vi "DestroyAllSessions.vi"(7 "DLL path":path, 8 "error in (no error)":errorcluster) -> (0 "error out":errorcluster)   [LabVIEW 2017, in "ONNX Class Library.lvlib"]
doc: "/**\n * @brief Уничтожить ВСЕ активные сессии (полная очистка памяти)\n * \n * Эта функция находит все созданные сессии в хранилище, освобождает их память,\n * удаляет метаданные и очищает список сессий. Полезно вызывать при завершении\n * работы приложения для гарантированного освобождения ресурсов.\n * \n * @return void\n * \n * @note После вызова все ранее полученные SessionID становятся невалидными\n * @note Не нужно вызывать DestroySession для каждой сессии отдельно\n * @note Безопасно вызывать, даже если сессий не было создано (ничего не сделает)\n */\nvoid DestroyAllSessions(void);"
uses:
  ONNX Class Library.lvlib
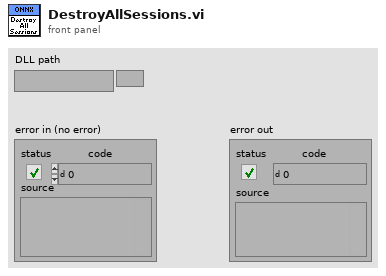
[diagram p1: front panel]
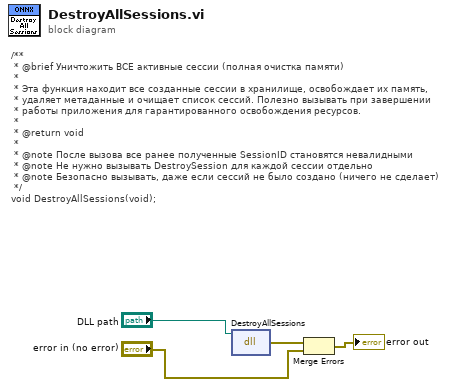
[diagram p0: block diagram]
diagram:
  # "/**\n * @brief Уничтожить ВСЕ активные сессии (полная очистка памяти)\n * \n * Эта функция находит все созданные сессии в хранилище, освобождает их память,\n * удаляет метаданные и очищает список сессий. Полезно вызывать при завершении\n * работы приложения для гарантированного освобождения ресурсов.\n * \n * @return void\n * \n * @note После вызова все ранее полученные SessionID становятся невалидными\n * @note Не нужно вызывать DestroySession для каждой сессии отдельно\n * @note Безопасно вызывать, даже если сессий не было создано (ничего не сделает)\n */\nvoid DestroyAllSessions(void);"
  n1 = dll-call lib="home/ivan/LabVIEWData/ONNX/Test/libonnx_wrapper/unix64/libonnx_wrapper.so" fn="DestroyAllSessions"(path in="DLL path") -> (error out=w4:errorcluster)  [unwired: 3 in, 1 out]
  n2 = Merge Errors(w4, "error in (no error)") -> (→"error out":errorcluster)
